vi "switch_line.vi"(0 "Node":dbl, 1 "event time":string="045", 2 "Event type":string="CL", 3 "Fault type (phases)":string="BC") -> (7 "Event switches":string caption="Result")   [LabVIEW 2020]
panel:
  in  "Evento?":bool
  # "CHAVEAMENTO DE  LINHA\nPOR FASES (A, B, C ou combinações)"
  # "E se não encontrar a fase?\nNão vai fazer nada! simulação SEM evento"
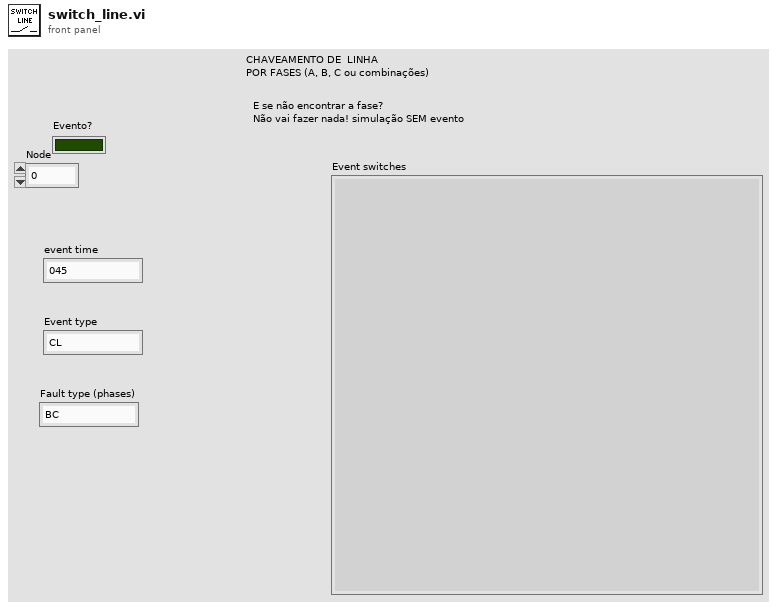
[diagram p1: front panel]
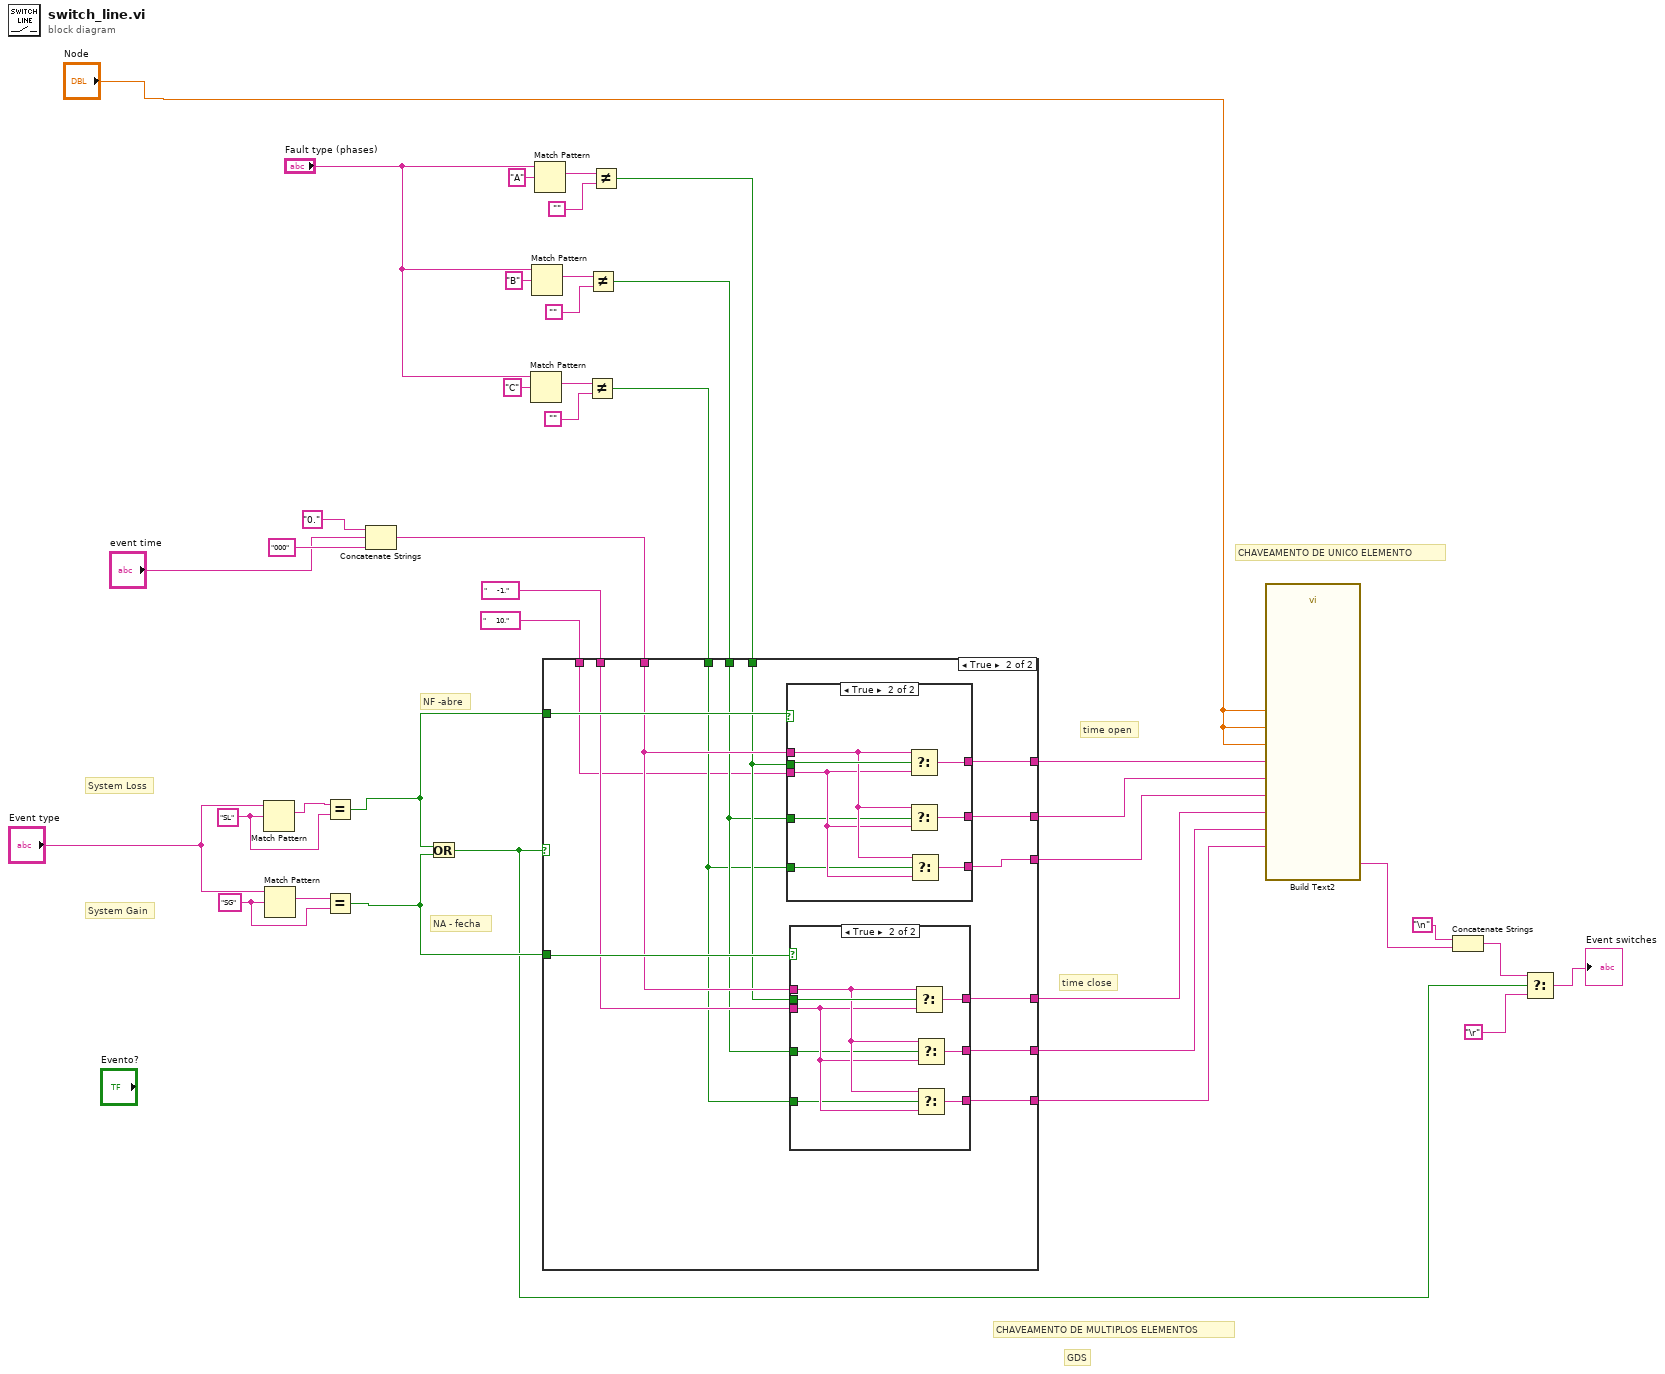
[diagram p0: block diagram]
diagram:
  w34 = "SL" ("regular expression")
  w35 = "SG" ("regular expression")
  # "time close"
  # "time open"
  # "GDS"
  # "CHAVEAMENTO DE MULTIPLOS ELEMENTOS"
  # "CHAVEAMENTO DE UNICO ELEMENTO"
  # "NA - fecha"
  # "NF -abre"
  # "System Gain"
  # "System Loss"
  n1 = Match Pattern(string="Event type", regular expression=w34) -> (match substring=w33:string)  [unwired: 1 in, 3 out]
  n2 = Match Pattern(string="Event type", regular expression=w35) -> (match substring=w37:string)  [unwired: 1 in, 3 out]
  n3 = Equal?(x=w33, y=w34) -> (x = y?=w28:bool)
  n4 = Equal?(x=w37, y=w35) -> (x = y?=w27:bool)
  n5 = Concatenate Strings("0." ("string"), "event time", "000" ("string")) -> (w29:string)
  n6 = Or(x=w28, y=w27) -> (x .or. y?=w26:bool)
  n7 = Match Pattern(string="Fault type (phases)", regular expression="C") -> (match substring=w15:string)  [unwired: 1 in, 3 out]
  n8 = Match Pattern(string="Fault type (phases)", regular expression="B") -> (match substring=w18:string)  [unwired: 1 in, 3 out]
  n9 = Match Pattern(string="Fault type (phases)", regular expression="A") -> (match substring=w21:string)  [unwired: 1 in, 3 out]
  n10 = Not Equal?(x=w15, y="") -> (x != y?=w10:bool)
  n11 = Not Equal?(x=w18, y="") -> (x != y?=w11:bool)
  n12 = Not Equal?(x=w21, y="") -> (x != y?=w12:bool)
  n13 = case shown="True" w26 {
    tunnel: w29 -> [_ w49]
    tunnel: "     -1." -> [w40 w50]
    tunnel: "     10." -> [w41 w42]
    tunnel: [w40 w48] -> w5
    tunnel: [w41 w55] -> w8
    tunnel: w27 -> [_ w51]
    tunnel: w28 -> [_ w54]
    tunnel: w12 -> [_ w47]
    tunnel: [w41 w53] -> w6
    tunnel: [w41 w52] -> w7
    tunnel: w11 -> [_ w46]
    tunnel: w10 -> [_ w45]
    tunnel: [w40 w44] -> w4
    tunnel: [w40 w43] -> w3
    frame False {
    }
    frame True {
      n14 = case shown="True" w54 {
        tunnel: [w65 w73] -> w55
        tunnel: w49 -> [_ w70]
        tunnel: w42 -> [w65 w69]
        tunnel: w47 -> [_ w72]
        tunnel: [w65 w71] -> w52
        tunnel: [w65 w68] -> w53
        tunnel: w46 -> [_ w67]
        tunnel: w45 -> [_ w66]
        frame False {
        }
        frame True {
          n15 = Select(t=w70, s=w72, f=w69) -> (s? t:f=w73:string)
          n16 = Select(t=w70, s=w67, f=w69) -> (s? t:f=w71:string)
          n17 = Select(t=w70, s=w66, f=w69) -> (s? t:f=w68:string)
        }
      }
      n18 = case shown="True" w51 {
        tunnel: w50 -> [w56 w61]
        tunnel: w49 -> [_ w62]
        tunnel: [w56 w64] -> w48
        tunnel: w47 -> [_ w63]
        tunnel: w46 -> [_ w60]
        tunnel: w45 -> [_ w59]
        tunnel: [w56 w58] -> w44
        tunnel: [w56 w57] -> w43
        frame False {
        }
        frame True {
          n19 = Select(t=w62, s=w63, f=w61) -> (s? t:f=w64:string)
          n20 = Select(t=w62, s=w60, f=w61) -> (s? t:f=w58:string)
          n21 = Select(t=w62, s=w59, f=w61) -> (s? t:f=w57:string)
        }
      }
    }
  }
  n22 = call "Build Text2"("inA_2"="Node", "time_close_A"=w5, "time_open_A"=w8, "inB_2"="Node", "time_close_B"=w4, "time_open_B"=w7, "inC_2"="Node", "time_close_C"=w3, "time_open_C"=w6) -> ("Result"=w2:string)  [unwired: 17 in, 1 out]
  n23 = Concatenate Strings("\n", w2) -> (w23:string)
  n24 = Select(t=w23, s=w26, f="\r") -> (s? t:f=→"Event switches":string)
